vi "sub_DegreesToRadians.vi"(11 "Angle (degrees)":dbl) -> (3 "Angle (Radians)":dbl)   [LabVIEW 2016, in "Project 2 LabVIEW.lvrbt"]
uses:
  Project 2 LabVIEW.lvrbt
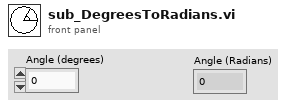
[diagram p1: front panel]
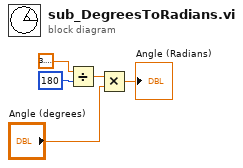
[diagram p0: block diagram]
diagram:
  n1 = Divide(x=3.141592653589793, y=180) -> (x/y=w3:dbl)
  n2 = Multiply(x=w3, y="Angle (degrees)") -> (x*y=→"Angle (Radians)":dbl)
